vi "解析参数预处理.vi"(1 "待解析参数内容":string) -> (0 "字符串":string)   [LabVIEW 2015]
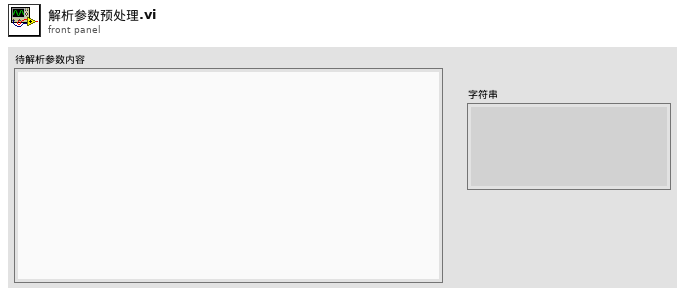
[diagram p1: front panel]
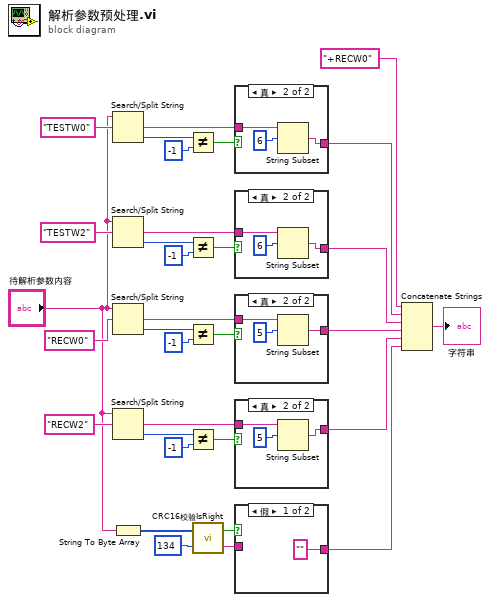
[diagram p0: block diagram]
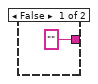
[diagram p3: hidden frame]
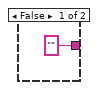
[diagram p4: hidden frame]
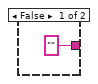
[diagram p5: hidden frame]
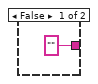
[diagram p6: hidden frame]
diagram:
  n1 = Search/Split String(string="待解析参数内容", search string/char (-)="TESTW0" ("帧首数据")) -> (match + rest of string=w19:string, offset of match=w18:i32)  [unwired: 1 in, 1 out]
  n2 = Search/Split String(string="待解析参数内容", search string/char (-)="TESTW2" ("帧首数据")) -> (match + rest of string=w16:string, offset of match=w15:i32)  [unwired: 1 in, 1 out]
  n3 = Search/Split String(string="待解析参数内容", search string/char (-)="RECW0" ("帧首数据")) -> (match + rest of string=w13:string, offset of match=w12:i32)  [unwired: 1 in, 1 out]
  n4 = Search/Split String(string="待解析参数内容", search string/char (-)="RECW2" ("帧首数据")) -> (match + rest of string=w7:string, offset of match=w23:i32)  [unwired: 1 in, 1 out]
  n5 = String To Byte Array(string="待解析参数内容") -> (unsigned byte array=w5:u8[])
  n6 = Not Equal?(x=w18, y=-1) -> (x != y?=w21:bool)
  n7 = Not Equal?(x=w15, y=-1) -> (x != y?=w17:bool)
  n8 = Not Equal?(x=w12, y=-1) -> (x != y?=w8:bool)
  n9 = Not Equal?(x=w23, y=-1) -> (x != y?=w9:bool)
  n10 = call "CRC16校验IsRight.vi"("含检验码数据长度"=u16 134 ("大小"), "输入数据"=w5) -> ("原始数据"=w2:string, "布尔"=w3:bool)
  n11 = case shown="真" w21 {
    tunnel: ["" ("待解析参数内容") w35] -> w20
    tunnel: w19 -> [_ w36]
    frame False {
    }
    frame True {
      n12 = String Subset(string=w36, offset (0)=6 ("偏移量(0)")) -> (substring=w35:string)  [unwired: 1 in]
    }
  }
  n13 = case shown="真" w17 {
    tunnel: ["" ("待解析参数内容") w39] -> w14
    tunnel: w16 -> [_ w40]
    frame False {
    }
    frame True {
      n14 = String Subset(string=w40, offset (0)=6 ("偏移量(0)")) -> (substring=w39:string)  [unwired: 1 in]
    }
  }
  n15 = case shown="真" w8 {
    tunnel: ["" ("待解析参数内容") w43] -> w11
    tunnel: w13 -> [_ w44]
    frame False {
    }
    frame True {
      n16 = String Subset(string=w44, offset (0)=5 ("偏移量(0)")) -> (substring=w43:string)  [unwired: 1 in]
    }
  }
  n17 = case shown="真" w9 {
    tunnel: ["" ("待解析参数内容") w47] -> w10
    tunnel: w7 -> [_ w48]
    frame False {
    }
    frame True {
      n18 = String Subset(string=w48, offset (0)=5 ("偏移量(0)")) -> (substring=w47:string)  [unwired: 1 in]
    }
  }
  n19 = case shown="假" w3 {
    tunnel: ["" ("待解析参数内容") w50] -> w1
    tunnel: w2 -> [_ w50]
    frame False {
    }
    frame True {
    }
  }
  n20 = Concatenate Strings("+RECW0" ("帧首数据"), w20, w14, w11, w10, w1) -> (→"字符串":string)
